vi "PSRR Monitor.vi"(0 "Exit":bool, 5 "Error Log":bool, 7 "Wait Time(sec)":i32) -> (4 "Error?":bool, 6 "Last Read PSRR (dB)":i32, 8 "Error Code":i32, 10 "Type":string, 12 "Description":string, 13 "Error Log Table":string[][](table), 14 "Obtained PSRR":i32(graph), 15 "Time":string)   [LabVIEW 2020]
doc: "This system is a Power Supply Rejection Ratio monitor which is used to get data from a PSRR and plot in a chart and give data about the error occurred."
uses:
  Typedefs/Stop cases.ctl
panel:
  out "Error out":errorcluster
  in  "Error in":errorcluster
  # "PSRR Monitor"
  # "Last Error Details"
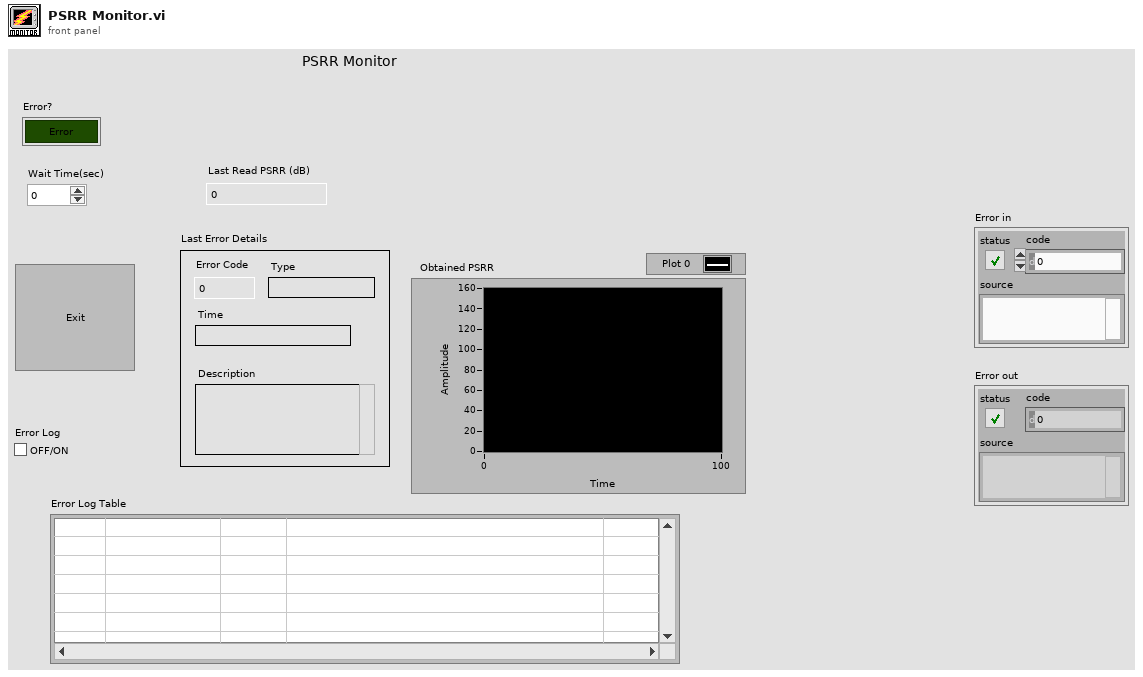
[diagram p1: front panel]
types:
  T1 = typedef "Stop cases.ctl" = enum16{"Initialize", "Write", "Stop"}
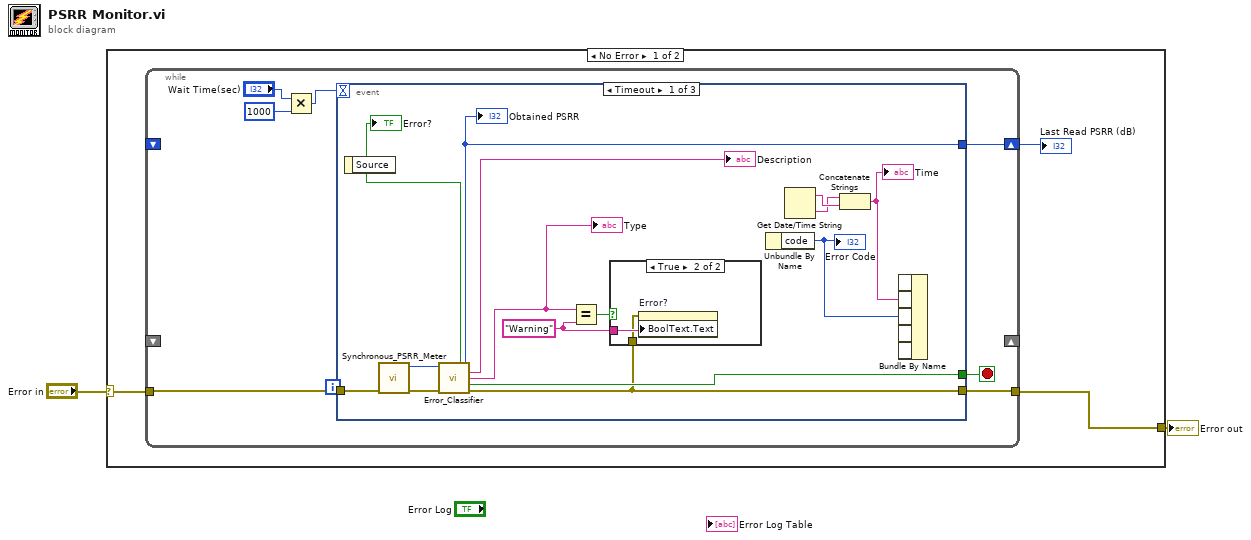
[diagram p0: block diagram]
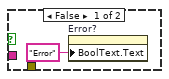
[diagram p2: hidden frame]
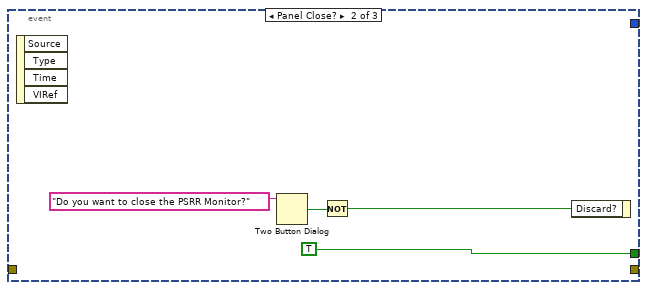
[diagram p3: hidden frame]
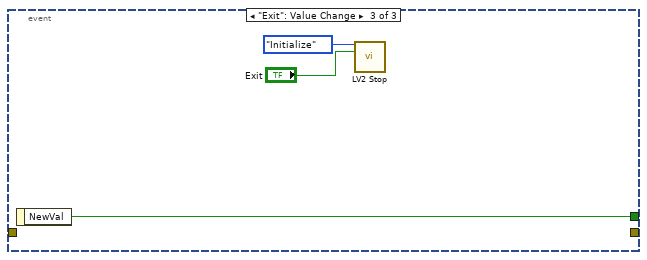
[diagram p4: hidden frame]
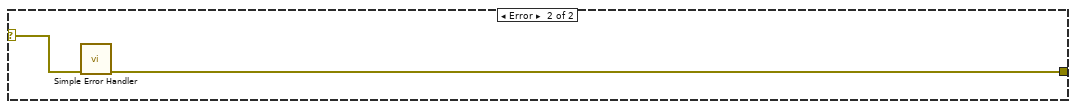
[diagram p5: hidden frame]
diagram:
  n1 = case shown="No Error" "Error in" {
    selector: "Error in" -> [w5 w39]
    tunnel: [w4 w38] -> w1
    frame No Error {
      n2 = while {
        tunnel: w5 -> [w7]
        tunnel: [w6] -> w4
        shift-right: [w8] -> w3
        shift-left: _ -> [_]
        shift-right: _ -> [_]
        shift-left: _ -> [_]
        stop <- w9 stop-if-true
        n3 = Multiply(x="Wait Time(sec)", y=1000) -> (x*y=w11:i32)
        n4 = event shown="[0] Timeout" {
          selector: _ -> [_ _ _]
          dyn-events: _ -> [_ _ _]
          timeout: w11 -> [_ _ _]
          tunnel: [w26 TRUE w37] -> w9
          tunnel: [w24 _ _] -> w8
          tunnel: w7 -> [w16 _ _]
          tunnel: [w13 _ _] -> w6
          event Timeout {
            w20 = "Warning" ("y")
            n5 = event-data() -> ()  [unwired: 1 in, 1 out]
            n6 = call "Synchronous_PSRR_Meter.vi"("error in"=w16) -> ("error out"=w15:errorcluster, "PSRR (dB)"=w27:i32)  [unwired: 9 in]
            n7 = call "Error_Classifier.vi"("PSRR"=w27, "Error in"=w15) -> ("Error?"=→"Error?":bool, "Waveform Chart"=w24:i32, "Description"=→"Description":string, "Type"=w14:string, "Stop"=w26:bool, "Error out"=w13:errorcluster)  [unwired: 8 in]
            "Obtained PSRR" <- w24
            "Type" <- w14
            n8 = Equal?(x=w14, y=w20) -> (x = y?=w25:bool)
            n9 = case shown="True" w25 {
              tunnel: w20 -> [_ w30]
              tunnel: w13 -> [_ w29]
              frame False {
                n10 = property on="Error?" class="Bool (strict)"("BoolText.Text"="Error" ("Boolean Text.Text")) -> ()  [unwired: 2 in, 2 out]
              }
              frame True {
                n11 = property on="Error?" class="Bool (strict)"(error in=w29, "BoolText.Text"=w30) -> ()  [unwired: 1 in, 2 out]
              }
            }
            n12 = Unbundle By Name() -> ("code"=w18:i32)  [unwired: 1 in]
            "Error Code" <- w18
            n13 = Get Date/Time String() -> (date string=w22:string, time string=w21:string)  [unwired: 3 in]
            n14 = Concatenate Strings(w21, w22) -> (w19:string)
            "Time" <- w19
            n15 = Bundle By Name(w19, w18) -> ()  [unwired: 4 in, 1 out]
          }
          event Panel Close? {
            n16 = event-data() -> ()  [unwired: 1 in, 4 out]
            n17 = Two Button Dialog(message="Do you want to close the PSRR Monitor?") -> (T button?=w33:bool)  [unwired: 2 in]
            n18 = Not(x=w33) -> (.not. x?=w34:bool)
            n19 = event-data("Discard?"=w34) -> ()  [unwired: 1 in, 1 out]
          }
          event "Exit": Value Change {
            n20 = event-data() -> ("NewVal"=w37:bool)  [unwired: 1 in]
            n21 = call "LV2 Stop.vi"("Operation"=Stop_cases."Initialize", "Stop"="Exit") -> ()  [unwired: 12 in, 2 out]
          }
        }
      }
      "Last Read PSRR (dB)" <- w3
    }
    frame Error {
      n22 = call <vilib>:"Simple Error Handler.vi"("error in (no error)"=w39) -> ("error out"=w38:errorcluster)  [unwired: 4 in, 4 out]
    }
  }
  "Error out" <- w1
